vi "Get cif_management_common_Channels.vi"(8 "error in (no error)":errorcluster, 11 "gRPCid":T1) -> (0 "error out":errorcluster, 2 "package_templatemessage":T2, 3 "gRPCid out":T1)   [LabVIEW 2021, in "CIFCoreChannel_server.lvlib"]
uses:
  CIFCoreChannel_server.lvlib
  cif_management_common_Channels.ctl
  cif_management_common_Channel.ctl
  cif_management_common_ChannelDirection.ctl
  cif_management_common_ChannelPattern.ctl
  <vilib>/gRPC/LabVIEW gRPC Library/Shared/grpcId.ctl
  cif_management_common_Channels_Flat.ctl
  cif_management_common_Channel_Flat.ctl
  2ed25e12-861d-4677-8ead-ace2906b2041.vi
  <vilib>/gRPC/LabVIEW gRPC Library/Shared/TranslateGrpcError.vi
  FlatToRichcif_management_common_Channel.vi
  <vilib>/gRPC/LabVIEW gRPC Library/Server API/Server/Get Server DLL Path.vi
  <vilib>/Utility/error.llb/Error Cluster From Error Code.vi
  <vilib>/gRPC/LabVIEW gRPC Library/grpc-lvsupport-release.lvlib
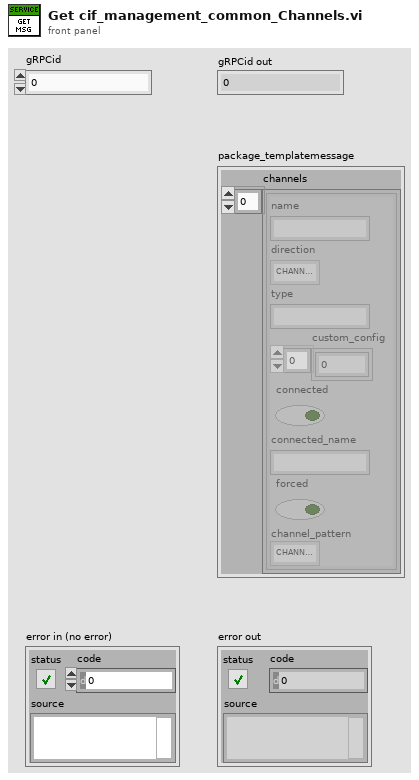
[diagram p1: front panel]
types:
  T1 = typedef "grpc-lvsupport-release.lvlib/grpcId.ctl" = u64
  T2 = typedef "CIFCoreChannel_server.lvlib/cif_management_common_Channels.ctl" = cluster{"channels":T3[]}
  T3 = typedef "CIFCoreChannel_server.lvlib/cif_management_common_Channel.ctl" = cluster{"name":string, "direction":T4, "type":string, "custom_config":u8[], "connected":bool, "connected_name":string, "forced":bool, "channel_pattern":T5}
  T4 = typedef "CIFCoreChannel_server.lvlib/cif_management_common_ChannelDirection.ctl" = enum32{"CHANNELDIRECTION_UNKNOWN", "CHANNELDIRECTION_PUBLISHER", "CHANNELDIRECTION_SUBSCRIBER"}
  T5 = typedef "CIFCoreChannel_server.lvlib/cif_management_common_ChannelPattern.ctl" = enum32{"CHANNELPATTERN_UNKNOWN", "CHANNELPATTERN_TAG", "CHANNELPATTERN_FIFO", "CHANNELPATTERN_MULTIFIFO", "CHANNELPATTERN_BACKPRESSUREFIFO"}
  T6 = typedef "CIFCoreChannel_server.lvlib/cif_management_common_Channels_Flat.ctl" = cluster{"channels":T7[]}
  T7 = typedef "CIFCoreChannel_server.lvlib/cif_management_common_Channel_Flat.ctl" = cluster{"name":string, "direction":T4, "type":string, "custom_config":u8[], "connected":bool, "connected_name":string, "forced":bool, "channel_pattern":T5}
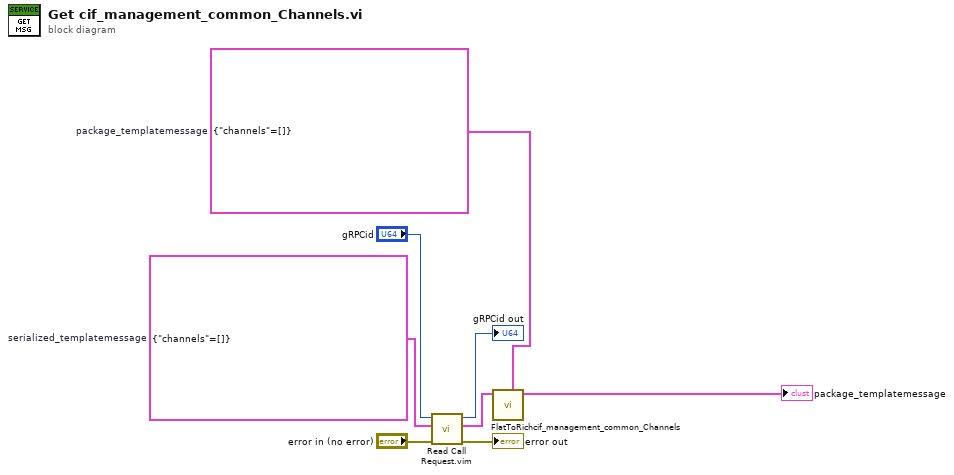
[diagram p0: block diagram]
diagram:
  w6 = T6 {"channels"=[]}  # serialized_templatemessage
  w5 = T2 {"channels"=[]}  # package_templatemessage
  n1 = call "Read Call Request.vim"("error in"="error in (no error)", "Request Type"=w6, "gRPCid in"="gRPCid") -> ("error out"=→"error out":errorcluster, "Request Data"=w4:T6, "gRPCid out"=→"gRPCid out":T1)  [unwired: 6 in]
  n2 = call "FlatToRichcif_management_common_Channels.vi"("OutputClusterType"=w5, "InputCluster"=w4) -> ("OutputCluster"=→"package_templatemessage":T2)  [unwired: 9 in]
